vi "New_file_CDH.vi"(0 "Sample name":string, 8 "Nota 3":string, 9 "Nota 2":string, 10 "Nota 01":string, 11 "File name":string) -> (3 "path":path)   [LabVIEW 2011]
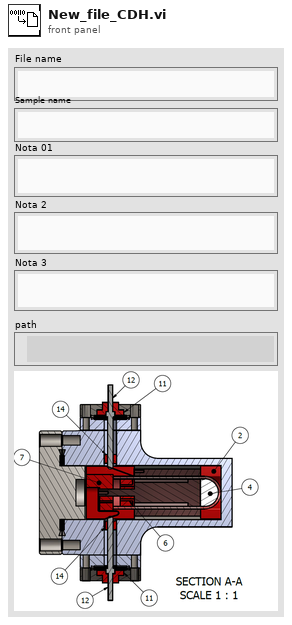
[diagram p1: front panel]
types:
  T1 = enum16{"open", "replace", "create", "open or create", "replace or create", "replace or create with confirmation"}
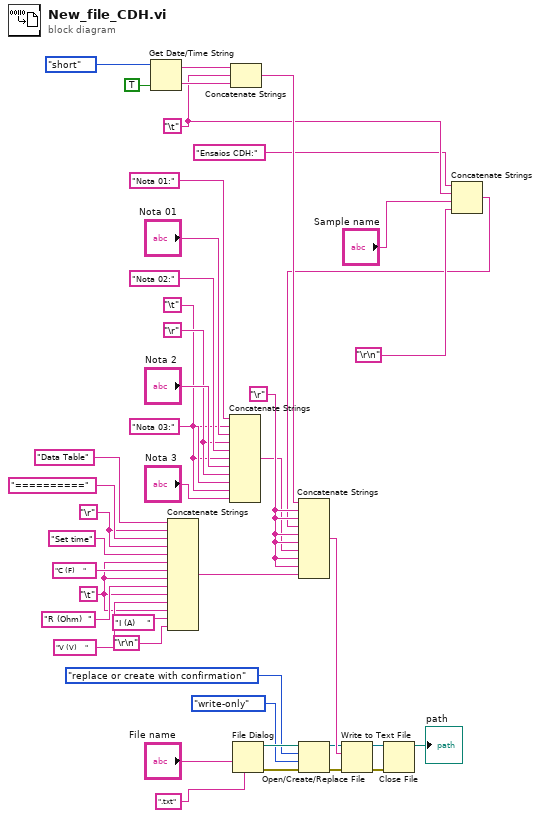
[diagram p0: block diagram]
diagram:
  w17 = "\t"
  w21 = "\r"
  w19 = "\t"
  w27 = "\r"
  w24 = "\r"
  w3 = "\t"
  n1 = Get Date/Time String(date format (0)=enum16{"short", "long", "abbreviated"}."short", want seconds? (F)=TRUE) -> (date string=w37:string, time string=w36:string)  [unwired: 1 in]
  n2 = Concatenate Strings("Data Table" ("string"), w27, "==========" ("string"), w27, "Set time" ("string"), w17, "C (F)    " ("string"), w17, "R (Ohm)  " ("string"), w17, "V (V)    " ("string"), w17, "I (A)    " ("string"), "\r\n") -> (w25:string)
  n3 = Concatenate Strings("Nota 01:" ("Nota 4"), w19, "Nota 01", w21, "Nota 02:" ("Nota 4"), w19, "Nota 2", w21, "Nota 03:" ("Nota 4"), w19, "Nota 3") -> (w18:string)
  n4 = Concatenate Strings(w37, w3, w36) -> (w26:string)
  n5 = File Dialog(6:".txt" ("pattern label"), 9:"File name") -> (0:w14:errorcluster, 3:w15:path)  [unwired: 2 in, 5 out]
  n6 = Open/Create/Replace File(file path (use dialog)=w15, error in=w14, operation (0:open)=T1."replace or create with confirmation", access (0:read/write)=enum16{"read/write", "read-only", "write-only"}."write-only") -> (refnum out=w11:refnum<file>, error out=w10:errorcluster)  [unwired: 3 out]
  n7 = Concatenate Strings("Ensaios CDH:" ("string"), w3, "Sample name", "\r\n") -> (w1:string)
  n8 = Concatenate Strings(w26, w24, w24, w1, w24, w24, w18, w24, w24, w25) -> (w35:string)
  n9 = Write to Text File(file (use dialog)=w11, text=w35, error in=w10) -> (refnum out=w9:refnum<file>, error out=w6:errorcluster)  [unwired: 1 in, 1 out]
  n10 = Close File(refnum=w9, error in=w6) -> (path=→"path":path)  [unwired: 1 out]
